vi "Monitor Stage.vi"(8 "error in (no error)":errorcluster, 11 "MAS in":refnum<class "MAS.lvclass">) -> (0 "error out":errorcluster, 3 "MAS out":refnum<class "MAS.lvclass">)   [LabVIEW 2022 SP3, in "MAS.lvclass"]
uses:
  MAS.lvclass
  iMotion Controller/iMotion Controller.lvclass
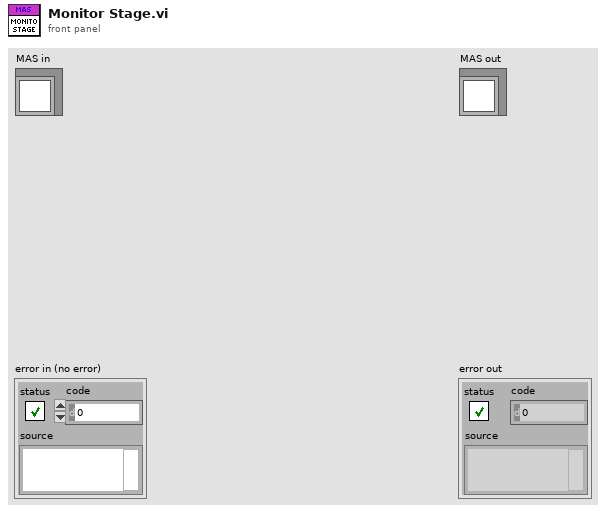
[diagram p1: front panel]
types:
  T1 = map{string, refnum<class "iMotion Controller.lvclass">}
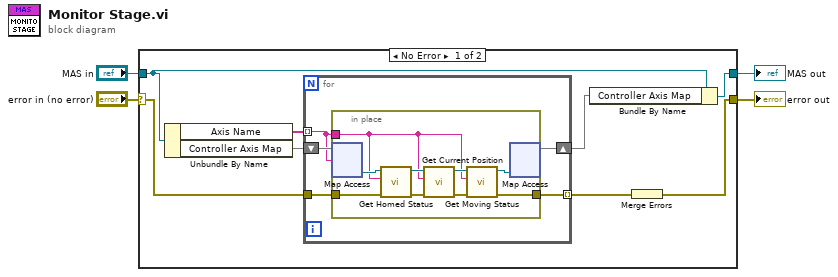
[diagram p0: block diagram]
diagram:
  n1 = case shown="No Error" "error in (no error)" {
    selector: "error in (no error)" -> [w9 w28]
    tunnel: [w7 w28] -> w3
    tunnel: [w6 w27] -> w1
    tunnel: "MAS in" -> [w12 w27]
    frame No Error {
      n2 = Unbundle By Name(w12) -> ("Axis Name"=w11:string[], "Controller Axis Map"=w10:T1)
      n3 = for {
        tunnel: w11 -> [w16] mode=indexing
        shift-right: [w15] -> w5
        shift-left: w10 -> [w17]
        tunnel: w9 -> [w14]
        tunnel: [w13] -> w8 mode=indexing
        n4 = in-place {
          in-place-border: w16 -> [w18]
          in-place-border: w14 -> [w26]
          in-place-border: [w21] -> w13
          n5 = in-place-map #1(w17, w16) -> (w25:refnum<class "iMotion Controller.lvclass">)  [unwired: 1 in, 1 out]
          n6 = call-dynamic "Get Homed Status.vi"("error in (no error)"=w26, 10:w18, "iMotion Controller in"=w25) -> ("error out"=w22:errorcluster, "iMotion Controller out"=w23:refnum<class "iMotion Controller.lvclass">)  [unwired: 6 in, 1 out]
          n7 = call-dynamic "Get Current Position.vi"("error in (no error)"=w22, 10:w18, "iMotion Controller in"=w23) -> ("error out"=w24:errorcluster, "iMotion Controller out"=w20:refnum<class "iMotion Controller.lvclass">)  [unwired: 6 in, 1 out]
          n8 = call-dynamic "Get Moving Status.vi"("error in (no error)"=w24, 10:w18, "iMotion Controller in"=w20) -> ("error out"=w21:errorcluster, "iMotion Controller out"=w19:refnum<class "iMotion Controller.lvclass">)  [unwired: 6 in, 1 out]
          n9 = in-place-map #1(w19) -> (w15:T1)  [unwired: 1 in, 2 out]
        }
      }
      n10 = Bundle By Name(cluster=w12, "Controller Axis Map"=w5) -> (w6:refnum<class "MAS.lvclass">)
      n11 = Merge Errors(w8) -> (w7:errorcluster)
    }
    frame Error {
    }
  }
  "error out" <- w3
  "MAS out" <- w1
